vi "statsCalc.vi"() -> ()   [LabVIEW 2014]
uses:
  <vilib>/gmath/statdist.llb/Normal Random.vi
  <userlib>/StatsCalculatorLabView/StatsCalculatorLabView.lvlib
  <vilib>/gmath/NI_Gmath.lvlib
  <vilib>/Analysis/NI_AALBase.lvlib
panel:
  out "Gaussian Distribution":T1(graph)
  out "Error State":errorcluster
  out "Standard Deviation":dbl(knob) scale=0.0..10.0
  out "Mean":dbl(knob) scale=0.0..10.0
  out "Sum":dbl(knob) scale=0.0..10.0
  in  "True\nStandard Deviation":dbl(knob)=0.5 scale=0.5..2.0
  in  "True Mean":dbl(knob) scale=-5.0..5.0
  in  "Number of Values":i32(knob)=50 scale=100.0..1000.0
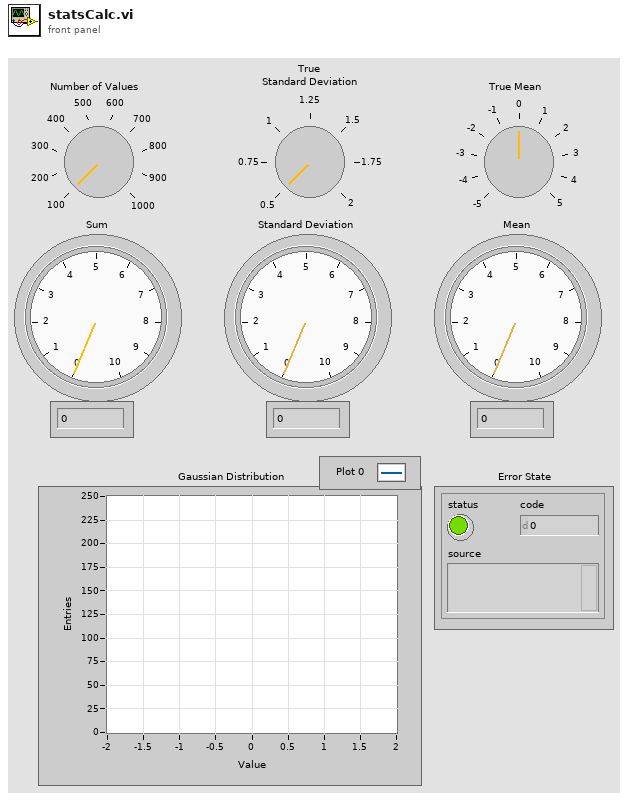
[diagram p1: front panel]
types:
  T1 = cluster{"X Values":dbl[], "Histogram: h(x)":i32[]}
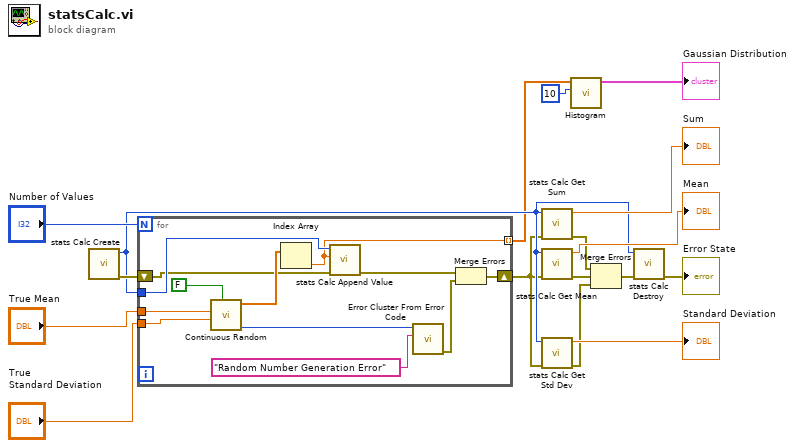
[diagram p0: block diagram]
diagram:
  n1 = call <userlib>:"stats Calc Create.vi"() -> ("error out"=w14:errorcluster, "function return"=w11:i32)  [unwired: 10 in]
  n2 = for {
    N: "Number of Values" -> [_]
    tunnel: w11 -> [w29]
    tunnel: "True\nStandard Deviation" -> [w28]
    tunnel: "True Mean" -> [w27]
    shift-right: [w19] -> w9
    shift-left: w14 -> [w22]
    tunnel: [w18] -> w3 mode=indexing
    n3 = call-poly <vilib>:"Continuous Random.vi"("reset"=FALSE, "std"=w28, "mean"=w27) -> ("error"=w24:i32, "normal random data"=w25:dbl[])  [unwired: 7 in]
    n4 = Index Array(array=w25) -> (element=w18:dbl)  [unwired: 1 in]
    n5 = call <userlib>:"stats Calc Append Value.vi"("error in (no error)"=w22, "value"=w18, "handle"=w29) -> ("error out"=w20:errorcluster)  [unwired: 8 in]
    n6 = call <vilib>:"Error Cluster From Error Code.vi"("error message (\"\")"="Random Number Generation Error", "error code (0)"=w24) -> ("error out"=w21:errorcluster)  [unwired: 7 in]
    n7 = Merge Errors(w20, w21) -> (w19:errorcluster)
  }
  n8 = call <userlib>:"stats Calc Get Sum.vi"("error in (no error)"=w9, "handle"=w11) -> ("error out"=w8:errorcluster, "function return"=→"Sum":dbl)  [unwired: 8 in]
  n9 = call <userlib>:"stats Calc Get Mean.vi"("error in (no error)"=w9, "handle"=w11) -> ("error out"=w7:errorcluster, "function return"=→"Mean":dbl)  [unwired: 8 in]
  n10 = call <userlib>:"stats Calc Get Std Dev.vi"("error in (no error)"=w9, "handle"=w11) -> ("error out"=w6:errorcluster, "function return"=→"Standard Deviation":dbl)  [unwired: 8 in]
  n11 = call <vilib>:"Histogram.vi"("intervals"=10, "X"=w3) -> ("Histogram Graph"=→"Gaussian Distribution":T1)  [unwired: 6 in, 3 out]
  n12 = Merge Errors(w8, w7, w6) -> (w5:errorcluster)
  n13 = call <userlib>:"stats Calc Destroy.vi"("error in (no error)"=w5, "handle"=w11) -> ("error out"=→"Error State":errorcluster)  [unwired: 9 in]
